vi "FTW-Endpoint-Receive.vi"(0 "FTW Endpoint":refnum<class "FTW-Endpoint-ZMQ.lvclass">, 5 "Timeout":i32 format="%dmsec", 11 "error in":errorcluster) -> (4 "FTW Endpoint out":refnum<class "FTW-Endpoint-ZMQ.lvclass">, 6 "Message Header":string, 8 "Message Body":string, 10 "Timed out?":bool, 15 "error out":errorcluster)   [LabVIEW 2012, in "FTW-Actor.lvlib" / "FTW-Endpoint-ZMQ.lvclass"]
uses:
  FTW-Endpoint-ZMQ.lvclass
  FTW-Endpoint-ZMQ.lvclass/FTW-Endpoint-ZMQ.ctl
panel:
  # "Inputs"
  # "Outputs"
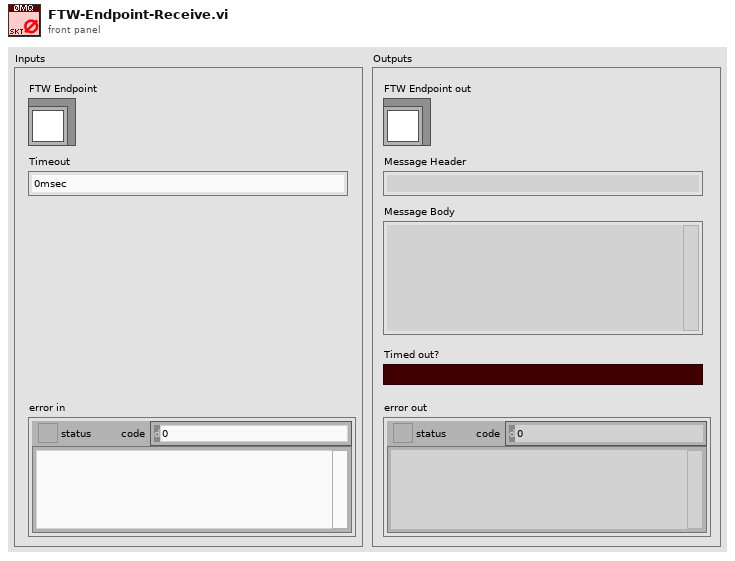
[diagram p1: front panel]
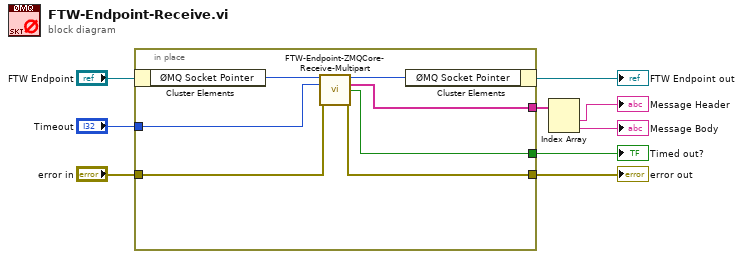
[diagram p0: block diagram]
diagram:
  n1 = in-place {
    in-place-border: "error in" -> [w16]
    in-place-border: "Timeout" -> [w13]
    in-place-border: [w12] -> w6
    in-place-border: [w11] -> w4
    in-place-border: [w10] -> w3
    n2 = in-place-cluster #1("FTW Endpoint") -> ("ØMQ Socket Pointer"=w15:u64)
    n3 = call "FTW-Endpoint-ZMQCore-Receive-Multipart.vi"("ØMQ Socket Pointer"=w15, "Timeout"=w13, "error in"=w16) -> ("ØMQ Socket Pointer out"=w14:u64, "Multipart Message"=w11:string[], "Timed out?"=w10:bool, "error out"=w12:errorcluster)  [unwired: 9 in]
    n4 = in-place-cluster #1("ØMQ Socket Pointer"=w14) -> (→"FTW Endpoint out":refnum<class "FTW-Endpoint-ZMQ.lvclass">)
  }
  "error out" <- w6
  "Timed out?" <- w3
  n5 = Index Array(array=w4) -> (element #1=→"Message Header":string, element #2=→"Message Body":string)  [unwired: 2 in]
